vi "Read.vi"(8 "error in (no error)":errorcluster, 11 "VISA resource name":refnum<visa-resource-name>) -> (0 "error out":errorcluster, 1 "Measurement Results":string[][](array[string]), 3 "VISA resource name out":refnum<visa-resource-name>)   [LabVIEW 2015, in "Voltech PM1000+.lvlib"]
doc: "Reads and returns a single measurement from the instrument."
uses:
  <instrlib>/Voltech PM1000+/Voltech PM1000+.lvlib
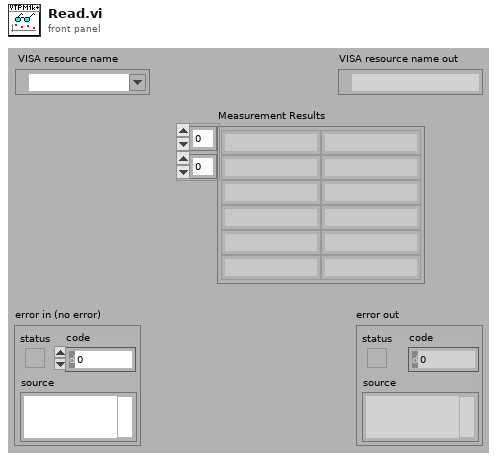
[diagram p1: front panel]
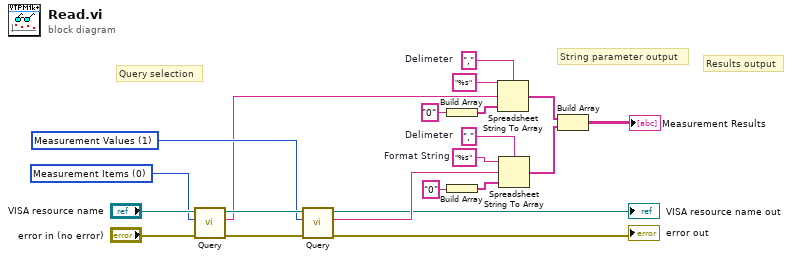
[diagram p0: block diagram]
diagram:
  w10 = ","  # Delimeter
  w14 = u16 1 items=["Measurement Items", "Measurement Values", "Blanking Setting", "Calibration Date", "Frequency Source", "Product ID", "Operating Mode", "Voltage Range", "Current Range", "Voltage Scaling Factor", "Current Scaling Factor", "Shunt Setting", "Auto Zero Setting"] ("Query")
  w17 = u16 0 items=["Measurement Items", "Measurement Values", "Blanking Setting", "Calibration Date", "Frequency Source", "Product ID", "Operating Mode", "Voltage Range", "Current Range", "Voltage Scaling Factor", "Current Scaling Factor", "Shunt Setting", "Auto Zero Setting"] ("Query")
  w18 = ","  # Delimeter
  w19 = "%s"  # Format String
  # "Results output"
  # "String parameter output"
  # "Query selection"
  n1 = call <instrlib>:"Query.vi"("error in (no error)"="error in (no error)", "Query"=w17, "VISA resource name"="VISA resource name") -> ("error out"=w15:errorcluster, "Result"=w8:string, "VISA resource name out"=w16:refnum<visa-resource-name>)  [unwired: 6 in]
  n2 = call <instrlib>:"Query.vi"("error in (no error)"=w15, "Query"=w14, "VISA resource name"=w16) -> ("error out"=→"error out":errorcluster, "Result"=w13:string, "VISA resource name out"=→"VISA resource name out":refnum<visa-resource-name>)  [unwired: 6 in]
  n3 = Build Array("0") -> (w6:string[])
  n4 = Build Array("0") -> (w5:string[])
  n5 = Spreadsheet String To Array(delimiter (Tab)=w10, format string="%s", spreadsheet string=w8, array type (2D Dbl)=w6) -> (array=w2:string[])
  n6 = Spreadsheet String To Array(delimiter (Tab)=w18, format string=w19, spreadsheet string=w13, array type (2D Dbl)=w5) -> (array=w3:string[])
  n7 = Build Array(w2, w3) -> (→"Measurement Results":string[][])
